vi "Array Status.vi"(7 "Action":T2(ring), 8 "error in":errorcluster, 9 "Position":cluster{"Row":i32, "Col":i32}, 10 "Display":refnum<vi>, 11 "semaphore":T1) -> (0 "error out":errorcluster)   [LabVIEW 2011]
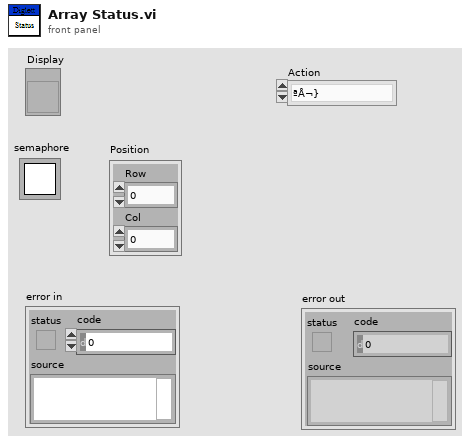
[diagram p1: front panel]
types:
  T1 = typedef "Semaphore RefNum" = refnum<k1>
  T2 = enum16{"ªÅ¬}", "¦a¹«¤É°_", "¦a¹«¤U­°", "¦a¹«³Q¥´", "¥´¿ù¬}"}
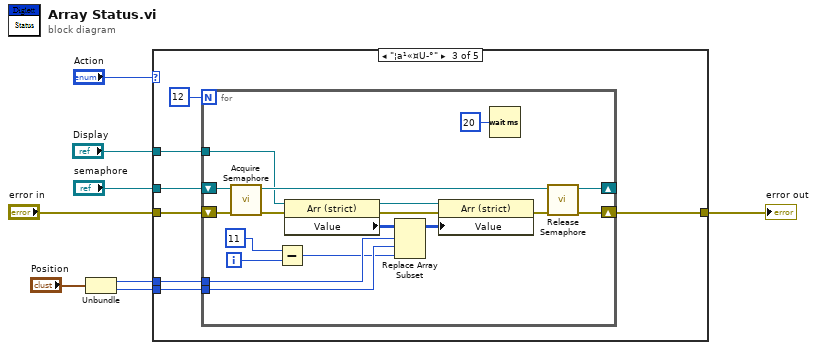
[diagram p0: block diagram]
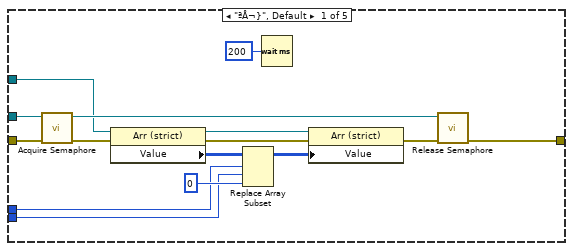
[diagram p2: hidden frame]
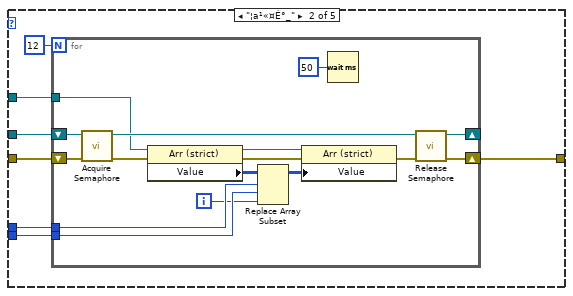
[diagram p3: hidden frame]
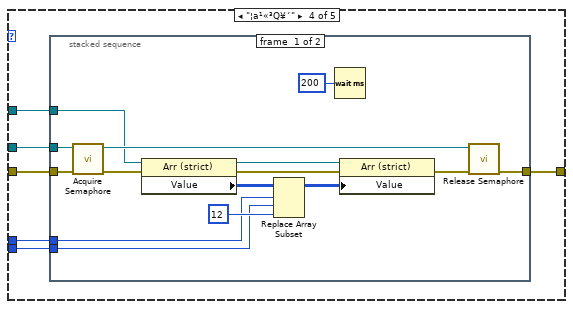
[diagram p4: hidden frame]
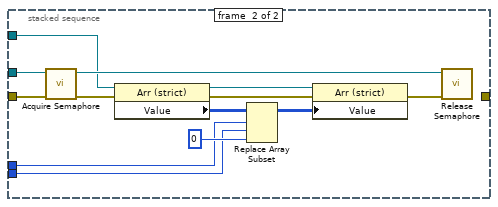
[diagram p5: hidden frame]
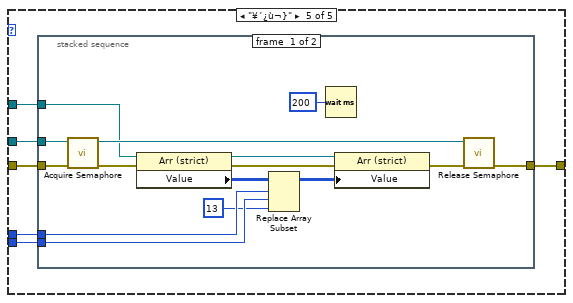
[diagram p6: hidden frame]
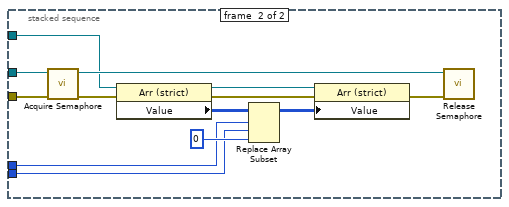
[diagram p7: hidden frame]
diagram:
  n1 = Unbundle("Position") -> ("Row"=w2:i32, "Col"=w1:i32)
  n2 = case shown="\"¦a¹«¤U­°\"" "Action" {
    tunnel: "error in" -> [w10 w29 w52 w75 w111]
    tunnel: [w9 w28 w51 w72 w109] -> w6
    tunnel: "semaphore" -> [w11 w27 w50 w74 w110]
    tunnel: "Display" -> [w12 w26 w49 w73 w108]
    tunnel: w2 -> [w13 w25 w48 w77 w107]
    tunnel: w1 -> [w14 w24 w47 w76 w106]
    frame "ªÅ¬}", Default {
      n3 = call <vilib>:"Acquire Semaphore.vi"("error in (no error)"=w10, "semaphore"=w11) -> ("error out"=w22:errorcluster, "semaphore out"=w23:T1)  [unwired: 3 in, 1 out]
      n4 = property class="Arr (strict)"(reference=w12, error in=w22) -> (reference out=w20:refnum<vi>, error out=w19:errorcluster, "Value"=w17:u16[][])
      n5 = Replace Array Subset(array=w17, new element=u16 0 ("Value"), index (row)=w13, index (col)=w14) -> (w16:u16[][])
      n6 = Wait (ms)(milliseconds to wait=u32 200) -> ()  [unwired: 1 out]
      n7 = property class="Arr (strict)"(reference=w20, error in=w19, "Value"=w16) -> (error out=w18:errorcluster)  [unwired: 1 out]
      n8 = call <vilib>:"Release Semaphore.vi"("error in (no error)"=w18, "semaphore"=w23) -> ("error out"=w9:errorcluster)  [unwired: 4 in, 1 out]
    }
    frame "¦a¹«¤É°_" {
      n9 = for {
        N: 12 -> [_]
        tunnel: w26 -> [w34]
        shift-right: [w44] -> w28
        shift-left: w29 -> [w45]
        shift-right: [w42] -> _
        shift-left: w27 -> [w43]
        tunnel: w25 -> [w33]
        tunnel: w24 -> [w32]
        i -> [w31]
        n10 = call <vilib>:"Acquire Semaphore.vi"("error in (no error)"=w45, "semaphore"=w43) -> ("error out"=w37:errorcluster, "semaphore out"=w35:T1)  [unwired: 3 in, 1 out]
        n11 = property class="Arr (strict)"(reference=w34, error in=w37) -> (reference out=w41:refnum<vi>, error out=w40:errorcluster, "Value"=w39:u16[][])
        n12 = Replace Array Subset(array=w39, new element=w31, index (row)=w33, index (col)=w32) -> (w38:u16[][])
        n13 = property class="Arr (strict)"(reference=w41, error in=w40, "Value"=w38) -> (error out=w36:errorcluster)  [unwired: 1 out]
        n14 = Wait (ms)(milliseconds to wait=u32 50) -> ()  [unwired: 1 out]
        n15 = call <vilib>:"Release Semaphore.vi"("error in (no error)"=w36, "semaphore"=w35) -> ("error out"=w44:errorcluster, "semaphore out"=w42:T1)  [unwired: 4 in]
      }
    }
    frame "¦a¹«¤U­°" {
      n16 = for {
        N: 12 -> [_]
        tunnel: w49 -> [w57]
        shift-right: [w69] -> w51
        shift-left: w52 -> [w70]
        shift-right: [w64] -> _
        shift-left: w50 -> [w67]
        tunnel: w48 -> [w56]
        tunnel: w47 -> [w55]
        i -> [w66]
        n17 = call <vilib>:"Acquire Semaphore.vi"("error in (no error)"=w70, "semaphore"=w67) -> ("error out"=w58:errorcluster, "semaphore out"=w68:T1)  [unwired: 3 in, 1 out]
        n18 = Subtract(x=11, y=w66) -> (x-y=w54:i32)
        n19 = property class="Arr (strict)"(reference=w57, error in=w58) -> (reference out=w63:refnum<vi>, error out=w62:errorcluster, "Value"=w61:u16[][])
        n20 = Replace Array Subset(array=w61, new element=w54, index (row)=w56, index (col)=w55) -> (w60:u16[][])
        n21 = property class="Arr (strict)"(reference=w63, error in=w62, "Value"=w60) -> (error out=w59:errorcluster)  [unwired: 1 out]
        n22 = Wait (ms)(milliseconds to wait=u32 20) -> ()  [unwired: 1 out]
        n23 = call <vilib>:"Release Semaphore.vi"("error in (no error)"=w59, "semaphore"=w68) -> ("error out"=w69:errorcluster, "semaphore out"=w64:T1)  [unwired: 4 in]
      }
    }
    frame "¦a¹«³Q¥´" {
      n24 = stacked-sequence {
        tunnel: w77 -> [w83 w94]
        tunnel: w76 -> [w82 w93]
        tunnel: w75 -> [w81 w95]
        tunnel: w74 -> [w80 w96]
        tunnel: w73 -> [w79 w97]
        tunnel: [w78 _] -> w72
        frame #0 {
          n25 = call <vilib>:"Acquire Semaphore.vi"("error in (no error)"=w81, "semaphore"=w80) -> ("error out"=w91:errorcluster, "semaphore out"=w92:T1)  [unwired: 3 in, 1 out]
          n26 = property class="Arr (strict)"(reference=w79, error in=w91) -> (reference out=w89:refnum<vi>, error out=w88:errorcluster, "Value"=w86:u16[][])
          n27 = Replace Array Subset(array=w86, new element=u16 12 ("Value"), index (row)=w83, index (col)=w82) -> (w85:u16[][])
          n28 = Wait (ms)(milliseconds to wait=u32 200) -> ()  [unwired: 1 out]
          n29 = property class="Arr (strict)"(reference=w89, error in=w88, "Value"=w85) -> (error out=w87:errorcluster)  [unwired: 1 out]
          n30 = call <vilib>:"Release Semaphore.vi"("error in (no error)"=w87, "semaphore"=w92) -> ("error out"=w78:errorcluster)  [unwired: 4 in, 1 out]
        }
        frame #1 {
          n31 = call <vilib>:"Acquire Semaphore.vi"("error in (no error)"=w95, "semaphore"=w96) -> ("error out"=w104:errorcluster, "semaphore out"=w105:T1)  [unwired: 3 in, 1 out]
          n32 = property class="Arr (strict)"(reference=w97, error in=w104) -> (reference out=w103:refnum<vi>, error out=w102:errorcluster, "Value"=w100:u16[][])
          n33 = Replace Array Subset(array=w100, new element=u16 0 ("Value"), index (row)=w94, index (col)=w93) -> (w99:u16[][])
          n34 = property class="Arr (strict)"(reference=w103, error in=w102, "Value"=w99) -> (error out=w101:errorcluster)  [unwired: 1 out]
          n35 = call <vilib>:"Release Semaphore.vi"("error in (no error)"=w101, "semaphore"=w105) -> ()  [unwired: 4 in, 2 out]
        }
      }
    }
    frame "¥´¿ù¬}" {
      n36 = stacked-sequence {
        tunnel: w111 -> [w124 w129]
        tunnel: w110 -> [w123 w130]
        tunnel: [w122 _] -> w109
        tunnel: w108 -> [w120 w131]
        tunnel: w107 -> [w114 w128]
        tunnel: w106 -> [w113 w127]
        frame #0 {
          n37 = call <vilib>:"Acquire Semaphore.vi"("error in (no error)"=w124, "semaphore"=w123) -> ("error out"=w125:errorcluster, "semaphore out"=w126:T1)  [unwired: 3 in, 1 out]
          n38 = property class="Arr (strict)"(reference=w120, error in=w125) -> (reference out=w119:refnum<vi>, error out=w118:errorcluster, "Value"=w116:u16[][])
          n39 = Replace Array Subset(array=w116, new element=u16 13 ("Value"), index (row)=w114, index (col)=w113) -> (w115:u16[][])
          n40 = Wait (ms)(milliseconds to wait=u32 200) -> ()  [unwired: 1 out]
          n41 = property class="Arr (strict)"(reference=w119, error in=w118, "Value"=w115) -> (error out=w117:errorcluster)  [unwired: 1 out]
          n42 = call <vilib>:"Release Semaphore.vi"("error in (no error)"=w117, "semaphore"=w126) -> ("error out"=w122:errorcluster)  [unwired: 4 in, 1 out]
        }
        frame #1 {
          n43 = call <vilib>:"Acquire Semaphore.vi"("error in (no error)"=w129, "semaphore"=w130) -> ("error out"=w138:errorcluster, "semaphore out"=w139:T1)  [unwired: 3 in, 1 out]
          n44 = property class="Arr (strict)"(reference=w131, error in=w138) -> (reference out=w137:refnum<vi>, error out=w136:errorcluster, "Value"=w134:u16[][])
          n45 = Replace Array Subset(array=w134, new element=u16 0 ("Value"), index (row)=w128, index (col)=w127) -> (w133:u16[][])
          n46 = property class="Arr (strict)"(reference=w137, error in=w136, "Value"=w133) -> (error out=w135:errorcluster)  [unwired: 1 out]
          n47 = call <vilib>:"Release Semaphore.vi"("error in (no error)"=w135, "semaphore"=w139) -> ()  [unwired: 4 in, 2 out]
        }
      }
    }
  }
  "error out" <- w6
